vi "HFRR ADV v03.vi"() -> ()   [LabVIEW 2025] (continued)
            n967 = File Dialog(6:"*.dgf" ("pattern"), 7:w2452, 11:w2437) -> (0:w2435:errorcluster, 3:w2443:path)  [unwired: 4 in, 2 out]
            n968 = Unbundle(w2435) -> ()  [unwired: 3 out]
            n969 = Path To String(path=w2443) -> (string=w2438:string)
            "string1 4" <- w2438
            n970 = Match Pattern(string=w2438, regular expression=".dgf" ("substring (\"\")")) -> (before substring=w2448:string)  [unwired: 1 in, 3 out]
            n971 = Concatenate Strings(w2448, ".duf" ("Substring")) -> (w2445:string)
            n972 = String To Path(string=w2445) -> (path=w2449:path)
            n973 = call <vilib>:"Read Characters From File.vi"("file path (dialog if empty)"=w2449, "start of read offset (chars.:0)"=60 ("start of read offset (chars.: 0)")) -> ("character string"=→"String Control 8":string)  [unwired: 4 in, 3 out]
            n974 = Strip Path(path=w2443) -> (name=w2441:string)  [unwired: 1 out]
            n975 = Match Pattern(string=w2441, regular expression=".dgf") -> (before substring=→"String Control 7":string)  [unwired: 1 in, 3 out]
          }
        }
        n976 = case shown="True" "OPEN 3" {
          frame False {
          }
          frame True {
            (unwired) 0  # existing file
            w2434 = "Choose a datalog file to open"  # prompt
            n977 = local write "OPEN 3"(FALSE ("OPEN 1")) -> ()
            n978 = String To Path(string="C:\\LAB-IQ-NXT\\Data\\") -> (path=w2419:path)
            n979 = File Dialog(6:"*.dgf" ("pattern"), 7:w2434, 11:w2419) -> (0:w2417:errorcluster, 3:w2425:path)  [unwired: 4 in, 2 out]
            n980 = Unbundle(w2417) -> ()  [unwired: 3 out]
            n981 = Path To String(path=w2425) -> (string=w2420:string)
            "string1 3" <- w2420
            n982 = Match Pattern(string=w2420, regular expression=".dgf" ("substring (\"\")")) -> (before substring=w2430:string)  [unwired: 1 in, 3 out]
            n983 = Concatenate Strings(w2430, ".duf" ("Substring")) -> (w2427:string)
            n984 = String To Path(string=w2427) -> (path=w2431:path)
            n985 = call <vilib>:"Read Characters From File.vi"("file path (dialog if empty)"=w2431, "start of read offset (chars.:0)"=60 ("start of read offset (chars.: 0)")) -> ("character string"=→"String Control 6":string)  [unwired: 4 in, 3 out]
            n986 = Strip Path(path=w2425) -> (name=w2423:string)  [unwired: 1 out]
            n987 = Match Pattern(string=w2423, regular expression=".dgf") -> (before substring=→"String Control 5":string)  [unwired: 1 in, 3 out]
          }
        }
        n988 = case shown="True" "OPEN 2" {
          frame False {
          }
          frame True {
            (unwired) 0  # existing file
            w2416 = "Choose a datalog file to open"  # prompt
            n989 = local write "OPEN 2"(FALSE ("OPEN 1")) -> ()
            n990 = String To Path(string="C:\\LAB-IQ-NXT\\Data\\") -> (path=w2401:path)
            n991 = File Dialog(6:"*.dgf" ("pattern"), 7:w2416, 11:w2401) -> (0:w2399:errorcluster, 3:w2407:path)  [unwired: 4 in, 2 out]
            n992 = Unbundle(w2399) -> ()  [unwired: 3 out]
            n993 = Path To String(path=w2407) -> (string=w2402:string)
            "string1 2" <- w2402
            n994 = Match Pattern(string=w2402, regular expression=".dgf" ("substring (\"\")")) -> (before substring=w2413:string)  [unwired: 1 in, 3 out]
            n995 = Concatenate Strings(w2413, ".duf" ("Substring")) -> (w2410:string)
            n996 = String To Path(string=w2410) -> (path=w2408:path)
            n997 = call <vilib>:"Read Characters From File.vi"("file path (dialog if empty)"=w2408, "start of read offset (chars.:0)"=60 ("start of read offset (chars.: 0)")) -> ("character string"=→"String Control 4":string)  [unwired: 4 in, 3 out]
            n998 = Strip Path(path=w2407) -> (name=w2405:string)  [unwired: 1 out]
            n999 = Match Pattern(string=w2405, regular expression=".dgf") -> (before substring=→"String Control 3":string)  [unwired: 1 in, 3 out]
          }
        }
        n1000 = case shown="True" "OPEN 1" {
          frame False {
          }
          frame True {
            (unwired) 0  # existing file
            w2398 = "Choose a datalog file to open"  # prompt
            n1001 = local write "OPEN 1"(FALSE ("OPEN 1")) -> ()
            n1002 = String To Path(string="C:\\LAB-IQ-NXT\\Data\\") -> (path=w2383:path)
            n1003 = File Dialog(6:"*.dgf" ("pattern"), 7:w2398, 11:w2383) -> (0:w2381:errorcluster, 3:w2389:path)  [unwired: 4 in, 2 out]
            n1004 = Unbundle(w2381) -> ()  [unwired: 3 out]
            n1005 = Path To String(path=w2389) -> (string=w2384:string)
            "string1" <- w2384
            n1006 = Match Pattern(string=w2384, regular expression=".dgf" ("substring (\"\")")) -> (before substring=w2394:string)  [unwired: 1 in, 3 out]
            n1007 = Concatenate Strings(w2394, ".duf" ("Substring")) -> (w2390:string)
            n1008 = String To Path(string=w2390) -> (path=w2395:path)
            n1009 = call <vilib>:"Read Characters From File.vi"("file path (dialog if empty)"=w2395, "start of read offset (chars.:0)"=60 ("start of read offset (chars.: 0)")) -> ("character string"=→"String Control 2":string)  [unwired: 4 in, 3 out]
            n1010 = Strip Path(path=w2389) -> (name=w2388:string)  [unwired: 1 out]
            n1011 = Match Pattern(string=w2388, regular expression=".dgf") -> (before substring=→"String Control":string)  [unwired: 1 in, 3 out]
          }
        }
        n1012 = case shown="True" "RSTV1 4" {
          frame False {
          }
          frame True {
            n1013 = property on="Stroke" class="XYGraph (strict)"("Y Scale.Display Format:Precision"=u8 2 ("Y Scale.Format & Precision:Precision")) -> ()  [unwired: 2 in, 2 out]
            n1014 = property on="Stroke" class="XYGraph (strict)"("X Scale.Range:Minimum"=0.0 ("Y Scale.Range:Maximum"), "X Scale.Range:Maximum"=75.0 ("X Scale.Range:Minimum"), "Y Scale.Range:Minimum"=0.98, "Y Scale.Range:Maximum"=1.02) -> ()  [unwired: 2 in, 2 out]
          }
        }
        n1015 = case shown="True" "rstv2" {
          frame False {
          }
          frame True {
            n1016 = property on="Coefficient Of Friction" class="XYGraph (strict)"("X Scale.Range:Minimum"=0.0 ("Y Scale.Range:Maximum"), "X Scale.Range:Maximum"=75.0, "Y Scale.Range:Minimum"=0.0, "Y Scale.Range:Maximum"=1.0 ("X Scale.Range:Minimum")) -> ()  [unwired: 2 in, 2 out]
            n1017 = property on="Coefficient Of Friction" class="XYGraph (strict)"("Y Scale.Display Format:Precision"=u8 3 ("Y Scale.Format & Precision:Precision")) -> ()  [unwired: 2 in, 2 out]
          }
        }
        n1018 = case shown="True" "RSTV1 3" {
          frame False {
          }
          frame True {
            n1019 = property on="Air Temperature" class="XYGraph (strict)"("X Scale.Range:Minimum"=0.0 ("Y Scale.Range:Minimum"), "X Scale.Range:Maximum"=75.0 ("Y Scale.Range:Maximum"), "Y Scale.Range:Minimum"=20.0 ("X Scale.Range:Minimum"), "Y Scale.Range:Maximum"=26.0 ("X Scale.Range:Maximum")) -> ()  [unwired: 2 in, 2 out]
            n1020 = property on="Air Temperature" class="XYGraph (strict)"("Y Scale.Display Format:Precision"=u8 2 ("Y Scale.Format & Precision:Precision")) -> ()  [unwired: 2 in, 2 out]
          }
        }
        n1021 = case shown="True" "RST CP" {
          frame False {
          }
          frame True {
            n1022 = property on="Sample Temperature" class="XYGraph (strict)"("X Scale.Range:Minimum"=0.0, "X Scale.Range:Maximum"=75.0, "Y Scale.Range:Minimum"=58.0, "Y Scale.Range:Maximum"=62.0) -> ()  [unwired: 2 in, 2 out]
            n1023 = property on="Sample Temperature" class="XYGraph (strict)"("Y Scale.Display Format:Precision"=u8 2 ("Y Scale.Format & Precision:Precision")) -> ()  [unwired: 2 in, 2 out]
          }
        }
        n1024 = case shown="True" "RST CP 2" {
          frame False {
          }
          frame True {
            n1025 = property on="XY Graph 13" class="XYGraph (strict)"("X Scale.Range:Minimum"=0.0, "X Scale.Range:Maximum"=75.0, "Y Scale.Range:Minimum"=0.0, "Y Scale.Range:Maximum"=100.0) -> ()  [unwired: 2 in, 2 out]
            n1026 = property on="XY Graph 13" class="XYGraph (strict)"("Y Scale.Display Format:Precision"=u8 0 ("Y Scale.Format & Precision:Precision")) -> ()  [unwired: 2 in, 2 out]
          }
        }
        n1027 = case shown="True" "RSTV1 2" {
          frame False {
          }
          frame True {
            n1028 = property on="Humidity" class="XYGraph (strict)"("X Scale.Range:Minimum"=0.0, "X Scale.Range:Maximum"=75.0, "Y Scale.Range:Minimum"=48.0, "Y Scale.Range:Maximum"=58.0) -> ()  [unwired: 2 in, 2 out]
            n1029 = property on="Humidity" class="XYGraph (strict)"("Y Scale.Display Format:Precision"=u8 0 ("Y Scale.Format & Precision:Precision")) -> ()  [unwired: 2 in, 2 out]
          }
        }
        n1030 = case shown="True" "RST CP 3" {
          frame False {
          }
          frame True {
            n1031 = property on="Air Temp vs Rh" class="XYGraph (strict)"("X Scale.Range:Minimum"=18.0, "X Scale.Range:Maximum"=28.0 ("X Scale.Range:Minimum"), "Y Scale.Range:Minimum"=30.0 ("X Scale.Range:Minimum"), "Y Scale.Range:Maximum"=70.0 ("X Scale.Range:Minimum")) -> ()  [unwired: 2 in, 2 out]
          }
        }
      }
      frame 2 {
        # "Elapsed time\ncof\nstroke\nmean pos\nTemp\nHumidity"
        n1032 = case shown="True" "Export" {
          frame False {
          }
          frame True {
            w2583 = "                                      " ("string")
            w2585 = "\r"
            (unwired) i16 6 ("width (-)")
            w2662 = "\r"
            w2594 = "\r"
            n1033 = local read "Sample ID"() -> (w2669:string)
            n1034 = local read "Temperature after test 2"() -> (w2656:dbl)
            n1035 = local read "Test Date"() -> (w2668:string)
            n1036 = local read "String 45"() -> (w2582:string)
            n1037 = local read "String 32"() -> (w2666:string)
            n1038 = local read "String 31"() -> (w2667:string)
            n1039 = local read "String 38"() -> (w2604:string)
            n1040 = local read "Humidity after test 2"() -> (w2652:dbl)
            n1041 = local read "s.NO"() -> (w2584:string)
            n1042 = local read "String 36"() -> (w2607:string)
            n1043 = local read "Temperature before test 2"() -> (w2651:dbl)
            n1044 = local read "String 37"() -> (w2610:string)
            n1045 = local read "AVP 2"() -> (w2649:dbl)
            n1046 = local read "HCF 2"() -> (w2660:dbl)
            n1047 = local read "MWSD 2"() -> (w2648:dbl)
            n1048 = local read "String 35"() -> (w2614:string)
            n1049 = local write "Export"(FALSE ("Export")) -> ()
            n1050 = local read "Humidity before test 2"() -> (w2637:dbl)
            n1051 = Concatenate Strings("7," ("string"), w2604) -> (w2605:string)
            n1052 = Concatenate Strings("6," ("string"), w2607) -> (w2608:string)
            n1053 = local read "S 39"() -> (w2615:string)
            n1054 = Concatenate Strings("5," ("string"), w2610) -> (w2611:string)
            n1055 = local read "String 34"() -> (w2619:string)
            n1056 = Concatenate Strings("4," ("string"), w2614) -> (w2613:string)
            n1057 = Concatenate Strings("3," ("string"), w2615) -> (w2617:string)
            n1058 = local read "S 38"() -> (w2622:string)
            n1059 = Number To Fractional String(number=w2660, width (-)=i16 6, precision (6)=i16 2) -> (F-format string=w2661:string)  [unwired: 1 in]
            n1060 = Number To Fractional String(number=w2648, width (-)=i16 6, precision (6)=i16 2) -> (F-format string=w2646:string)  [unwired: 1 in]
            n1061 = Number To Fractional String(number=w2649, width (-)=i16 6, precision (6)=i16 2) -> (F-format string=w2647:string)  [unwired: 1 in]
            n1062 = Number To Fractional String(number=w2656, width (-)=i16 6, precision (6)=i16 2) -> (F-format string=w2655:string)  [unwired: 1 in]
            n1063 = Number To Fractional String(number=w2652, width (-)=i16 6, precision (6)=i16 2) -> (F-format string=w2650:string)  [unwired: 1 in]
            n1064 = Number To Fractional String(number=w2651, width (-)=i16 6, precision (6)=i16 2) -> (F-format string=w2657:string)  [unwired: 1 in]
            n1065 = Number To Fractional String(number=w2637, width (-)=i16 6, precision (6)=i16 2) -> (F-format string=w2636:string)  [unwired: 1 in]
            n1066 = local read "String 39"() -> (w2601:string)
            n1067 = Concatenate Strings("2," ("string"), w2619) -> (w2618:string)
            n1068 = local read "WS1.4 2"() -> (w2664:dbl)
            n1069 = Concatenate Strings(w2594, "," ("string"), w2582, w2584, w2583, w2666, w2669, w2583, w2667, w2668, w2594) -> (w2592:string)
            n1070 = Concatenate Strings("1," ("string"), w2622) -> (w2621:string)
            n1071 = Concatenate Strings("8," ("string"), w2601) -> (w2602:string)
            n1072 = Number To Fractional String(number=w2664, precision (6)=i16 2) -> (F-format string=w2665:string)  [unwired: 2 in]
            n1073 = Concatenate Strings(w2662, w2621, w2636, w2662, w2618, w2657, w2662, w2617, w2650, w2662, w2613, w2655, w2662, w2611, w2646, w2662, w2608, w2647, w2662, w2605, w2661, w2662, w2602, w2665) -> (w2624:string)
            n1074 = Concatenate Strings("S.No," ("string"), "                                       Parameters" ("string")) -> (w2595:string)
            n1075 = local read "TITTLE"() -> (w2590:string)
            n1076 = local read "String 33"() -> (w2599:string)
            n1077 = local read "Tested by"() -> (w2598:string)
            n1078 = Concatenate Strings("=" ("string"), w2590) -> (w2589:string)
            n1079 = local read "String 29"() -> (w2631:string)
            n1080 = Concatenate Strings("," ("string"), "                                                                             " ("string")) -> (w2587:string)
            n1081 = Concatenate Strings(w2589, w2585, w2592, w2585, w2595, w2624, w2585, w2587, w2599, w2598) -> (→"export":string)
            n1082 = Match Pattern(string=w2631, regular expression=".dwm") -> (before substring=w2627:string)  [unwired: 1 in, 3 out]
            "before substring" <- w2627
            n1083 = case shown="\"xlx\"" "Select File Type" {
              tunnel: w2627 -> [w2672 w2674 w2676]
              tunnel: [w2670 w2675 w2677] -> w2626
              frame "xlx" {
                n1084 = Concatenate Strings(w2672, ".xls" ("string")) -> (w2670:string)
              }
              frame "csv" {
                n1085 = Concatenate Strings(w2674, ".csv" ("string")) -> (w2675:string)
              }
              frame "txt" {
                n1086 = Concatenate Strings(w2676, ".txt" ("string")) -> (w2677:string)
              }
            }
            n1087 = String To Path(string=w2626) -> (path=w2633:path)
            n1088 = local read "export"() -> (w2628:string)
            n1089 = call <vilib>:"Write Characters To File.vi"("append to file? (new file:F)"=FALSE, "character string"=w2628, "file path (dialog if empty)"=w2633) -> ()  [unwired: 2 in, 1 out]
          }
        }
        n1090 = case shown="True" "OK Button 16" {
          frame False {
          }
          frame True {
            n1091 = stacked-sequence {
              frame #0 {
                n1092 = local read "Numeric 16"() -> (w2792:i32)
                n1093 = local write "Numeric 10"(w2792) -> ()
              }
              frame #1 {
                n1094 = local read "String 29"() -> (w2796:string)
                n1095 = String To Path(string=w2796) -> (path=w2795:path)
                n1096 = local read "S.NO"() -> (→"s.NO":string)
                n1097 = Open/Create/Replace File "Open File"(file path (use dialog)=w2795) -> (refnum out=w2797:refnum<file>)  [unwired: 5 in, 2 out]
                n1098 = for {
                  N: 16 -> [_]
                  tunnel: w2797 -> [w2804]
                  i -> [w2800]
                  (unwired) TRUE ("line mode (F)")
                  n1099 = Read from Text File "Read File"(file (use dialog)=w2804) -> (text=w2798:string)  [unwired: 3 in, 3 out]
                  n1100 = Match Pattern(string=w2798, regular expression="(") -> (after substring=w2803:string)  [unwired: 1 in, 3 out]
                  n1101 = Match Pattern(string=w2803, regular expression=")") -> (before substring=w2799:string)  [unwired: 1 in, 3 out]
                  n1102 = case shown="1" w2800 {
                    tunnel: w2799 -> [w2805 w2806 _ _ w2807 w2808 w2809 w2811 w2813 w2815 w2817 w2819 w2821 w2823 _]
                    tunnel: w2798 -> [_ _ _ _ _ _ _ _ _ _ _ _ _ _ _]
                    frame 0 {
                      "TITTLE" <- w2805
                    }
                    frame 1 {
                      "Sample ID" <- w2806
                    }
                    frame 2 {
                    }
                    frame 3 {
                    }
                    frame 4 {
                      "Test Date" <- w2807
                    }
                    frame 5 {
                      "Tested by" <- w2808
                    }
                    frame 6 {
                      n1103 = Fract/Exp String To Number(string=w2809) -> (number=→"Humidity before test 2":dbl)  [unwired: 3 in, 1 out]
                    }
                    frame 7 {
                      n1104 = Fract/Exp String To Number(string=w2811) -> (number=→"Temperature before test 2":dbl)  [unwired: 3 in, 1 out]
                    }
                    frame 8 {
                      n1105 = Fract/Exp String To Number(string=w2813) -> (number=→"Humidity after test 2":dbl)  [unwired: 3 in, 1 out]
                    }
                    frame 9 {
                      n1106 = Fract/Exp String To Number(string=w2815) -> (number=→"Temperature after test 2":dbl)  [unwired: 3 in, 1 out]
                    }
                    frame 10 {
                      n1107 = Fract/Exp String To Number(string=w2817) -> (number=→"MWSD 2":dbl)  [unwired: 3 in, 1 out]
                    }
                    frame 11 {
                      n1108 = Fract/Exp String To Number(string=w2819) -> (number=→"AVP 2":dbl)  [unwired: 3 in, 1 out]
                    }
                    frame 12 {
                      n1109 = Fract/Exp String To Number(string=w2821) -> (number=→"HCF 2":dbl)  [unwired: 3 in, 1 out]
                    }
                    frame 13 {
                      n1110 = Fract/Exp String To Number(string=w2823) -> (number=→"WS1.4 2":dbl)  [unwired: 3 in, 1 out]
                    }
                    frame 14, Default {
                    }
                  }
                }
              }
              frame #2 {
              }
            }
            n1111 = local write "OK Button 16"(FALSE ("OK Button 13")) -> ()
          }
        }
        n1112 = call <vilib>:"Query Available Printers.vi"() -> ("system configured printers"=w2467:string[])  [unwired: 9 in, 2 out]
        "System Configured Printers 2" <- w2467
        n1113 = Index Array(array=w2467, index="Select Printer 3") -> (element=w2469:string)
        "Selected Printer" <- w2469
        n1114 = local read "OK Button 16"() -> (w2463:bool)
        n1115 = case shown="True" "Print" {
          tunnel: w2469 -> [_ w2761]
          frame False {
          }
          frame True {
            (unwired) i16 6 ("width (-)")
            (unwired) "TESTED BY : "
            (unwired) "TESTED DATE :"
            (unwired) "SAMPLE ID : "
            (unwired) "SAMPLE DESIGN : "
            w2719 = "\r"
            w2736 = "\r"
            # "add image"
            n1116 = local read "String 45"() -> (w2679:string)
            n1117 = local read "Sample ID"() -> (w2709:string)
            n1118 = local read "Tested by"() -> (w2712:string)
            n1119 = local read "Test Date"() -> (w2710:string)
            n1120 = local read "String 32"() -> (w2714:string)
            n1121 = local read "String 31"() -> (w2713:string)
            n1122 = local read "String 33"() -> (w2715:string)
            n1123 = local read "s.NO"() -> (w2680:string)
            n1124 = call <vilib>:"New Report.vi"("report type"=enum16{"Standard Report", "HTML"}."Standard Report") -> ("report out"=w2759:refnum<class "NI_report.lvclass">, "error out"=w2758:errorcluster)  [unwired: 13 in]
            n1125 = local read "TITTLE"() -> (w2711:string)
            n1126 = call-dynamic "Set Report Header Text.vi"("report in"=w2759, "center header text"=w2711, "error in (no error)"=w2758) -> ("report out"=w2730:refnum<class "NI_report.lvclass">, "error out"=w2731:errorcluster)  [unwired: 11 in]
            n1127 = Concatenate Strings(w2736, w2679, w2680, w2736, w2714, w2709, w2736, w2713, w2710, w2736, w2715, w2712, w2736) -> (w2729:string)
            "test by" <- w2729
            n1128 = local read "Temperature after test 2"() -> (w2725:dbl)
            n1129 = local read "String 38"() -> (w2685:string)
            n1130 = local read "Humidity after test 2"() -> (w2734:dbl)
            n1131 = local read "String 36"() -> (w2689:string)
            n1132 = local read "Temperature before test 2"() -> (w2735:dbl)
            n1133 = local read "String 37"() -> (w2692:string)
            n1134 = local read "AVP 2"() -> (w2738:dbl)
            n1135 = local read "HCF 2"() -> (w2721:dbl)
            n1136 = local read "MWSD 2"() -> (w2739:dbl)
            n1137 = local read "String 35"() -> (w2694:string)
            n1138 = call-poly <vilib>:"Append Report Text.vi"("report in"=w2730, "text"=w2729, "error in (no error)"=w2731) -> ("report out"=w2733:refnum<class "NI_report.lvclass">, "error out"=w2732:errorcluster)  [unwired: 9 in, 2 out]
            n1139 = local read "Humidity before test 2"() -> (w2750:dbl)
            n1140 = Concatenate Strings("7)" ("string"), w2685) -> (w2686:string)
            n1141 = local read "S 39"() -> (w2697:string)
            n1142 = local read "String 34"() -> (w2699:string)
            n1143 = Concatenate Strings("6)" ("string"), w2689) -> (w2688:string)
            n1144 = Concatenate Strings("5)" ("string"), w2692) -> (w2691:string)
            n1145 = Concatenate Strings("4)" ("string"), w2694) -> (w2695:string)
            n1146 = Concatenate Strings("3)" ("string"), w2697) -> (w2698:string)
            n1147 = local read "S 38"() -> (w2704:string)
            n1148 = Concatenate Strings("2)" ("string"), w2699) -> (w2700:string)
            n1149 = Number To Fractional String(number=w2721, width (-)=i16 6, precision (6)=i16 2) -> (F-format string=w2720:string)  [unwired: 1 in]
            n1150 = Number To Fractional String(number=w2739, width (-)=i16 6, precision (6)=i16 2) -> (F-format string=w2741:string)  [unwired: 1 in]
            n1151 = Number To Fractional String(number=w2738, width (-)=i16 6, precision (6)=i16 2) -> (F-format string=w2740:string)  [unwired: 1 in]
            n1152 = Number To Fractional String(number=w2725, width (-)=i16 6, precision (6)=i16 2) -> (F-format string=w2726:string)  [unwired: 1 in]
            n1153 = Number To Fractional String(number=w2734, width (-)=i16 6, precision (6)=i16 2) -> (F-format string=w2737:string)  [unwired: 1 in]
            n1154 = Number To Fractional String(number=w2735, width (-)=i16 6, precision (6)=i16 2) -> (F-format string=w2724:string)  [unwired: 1 in]
            n1155 = Number To Fractional String(number=w2750, width (-)=i16 6, precision (6)=i16 2) -> (F-format string=w2755:string)  [unwired: 1 in]
            n1156 = call-poly <vilib>:"Append Report Text.vi"("report in"=w2733, "error in (no error)"=w2732) -> ("report out"=w2754:refnum<class "NI_report.lvclass">, "error out"=w2752:errorcluster)  [unwired: 10 in, 2 out]
            n1157 = local read "String 39"() -> (w2682:string)
            n1158 = local read "WS1.4 2"() -> (w2717:dbl)
            n1159 = Concatenate Strings("1)" ("string"), w2704) -> (w2703:string)
            n1160 = Concatenate Strings("8)" ("string"), w2682) -> (w2683:string)
            n1161 = Number To Fractional String(number=w2717, precision (6)=i16 2) -> (F-format string=w2716:string)  [unwired: 2 in]
            n1162 = Concatenate Strings(w2719, w2703, w2755, w2719, w2700, w2724, w2719, w2698, w2737, w2719, w2695, w2726, w2719, w2691, w2741, w2719, w2688, w2740, w2719, w2686, w2720, w2719, w2683, w2716) -> (w2707:string)
            "export 2" <- w2707
            n1163 = call-poly <vilib>:"Append Report Text.vi"("report in"=w2754, "text"=w2707, "error in (no error)"=w2752) -> ("report out"=w2753:refnum<class "NI_report.lvclass">, "error out"=w2751:errorcluster)  [unwired: 9 in, 2 out]
            n1164 = call-dynamic "Print Report.vi"("report in"=w2753, "printer name (default)"=w2761, "error in (no error)"=w2751) -> ("report out"=w2763:refnum<class "NI_report.lvclass">, "error out"=w2764:errorcluster)  [unwired: 11 in]
            n1165 = local read "test by"() -> (w2706:string)
            n1166 = local read "TITTLE"() -> (w2708:string)
            n1167 = local write "Print"(FALSE ("Print FF")) -> ()
            n1168 = call-dynamic "Dispose Report.vi"("report in"=w2763, "error in (no error)"=w2764) -> ()  [unwired: 13 in, 1 out]
            n1169 = Concatenate Strings(w2708, w2707, w2706) -> (→"output":string)
          }
        }
        n1170 = case shown="True" w2463 {
          frame False {
          }
          frame True {
            n1171 = flat-sequence {
              frame #0 {
              }
              frame #1 {
                n1172 = Wait (ms)(milliseconds to wait=u32 100) -> ()  [unwired: 1 out]
              }
              frame #2 {
                n1173 = local write "OK Button 16"(FALSE ("Print 3")) -> ()
              }
            }
          }
        }
        n1174 = case shown="True" "OK Button 17" {
          frame False {
          }
          frame True {
            (unwired) 0  # existing file
            w2778 = "Choose a datalog file to open"  # prompt
            n1175 = local read "String"() -> (w2773:string)
            n1176 = local write "OK Button 17"(FALSE ("OK Button 17")) -> ()
            n1177 = String To Path(string=w2773) -> (path=w2774:path)
            n1178 = File Dialog(6:"*.duf" ("pattern"), 7:w2778, 11:w2774) -> (0:w2765:errorcluster, 3:w2784:path)  [unwired: 4 in, 2 out]
            n1179 = Unbundle(w2765) -> ()  [unwired: 3 out]
            n1180 = Open/Create/Replace File "Open File"(file path (use dialog)=w2784) -> (refnum out=w2776:refnum<file>)  [unwired: 5 in, 2 out]
            n1181 = Path To String(path=w2784) -> (string=w2767:string)
            n1182 = while {
              tunnel: w2776 -> [w2788]
              i -> [w2785]
              stop <- w2786 continue-if-true
              (unwired) TRUE ("line mode (F)")
              n1183 = local write "Numeric 16"(w2785) -> ()
              n1184 = Read from Text File "Read File"(file (use dialog)=w2788) -> (text=w2787:string)  [unwired: 3 in, 3 out]
              n1185 = String Length(string=w2787) -> (length=w2790:i32)
              n1186 = Greater?(x=w2790, y=1) -> (0:w2786:bool)
            }
            n1187 = local write "String 29"(w2767) -> ()
            n1188 = Match Pattern(string=w2767, regular expression=".dwm" ("substring (\"\")")) -> (before substring=w2768:string)  [unwired: 1 in, 3 out]
            "String Indicator 3" <- w2768
            n1189 = Search and Replace String(input string=w2767, search string=".duf", replace string=".dgf" ("replace string (\"\")")) -> (result string=→"String Indicator 4":string)  [unwired: 5 in, 3 out]
            n1190 = String To Path(string=w2768) -> (path=w2775:path)
            "path" <- w2775
            n1191 = Strip Path(path=w2784) -> (name=w2782:string)  [unwired: 1 out]
            n1192 = call <vilib>:"Read Characters From File.vi"("file path (dialog if empty)"=w2775, "start of read offset (chars.:0)"=60 ("start of read offset (chars.: 0)")) -> ("character string"=→"String Indicator 2":string)  [unwired: 4 in, 3 out]
            n1193 = Match Pattern(string=w2782, regular expression=".dwm") -> (before substring=w2766:string)  [unwired: 1 in, 3 out]
            "String Indicator" <- w2766
            n1194 = local write "TITTLE 2"(w2766) -> ()
          }
        }
        n1195 = case shown="True" "Print 2" {
          frame False {
          }
          frame True {
            n1196 = flat-sequence {
              frame #0 {
                n1197 = local read "Ref A Test Date :"() -> (→"TITTLE 4":string)
                n1198 = local read "Sample ID"() -> (→"Sample ID  2":string)
                n1199 = local read "s.NO"() -> (→"s.NO 2":string)
                n1200 = local read "Test Date"() -> (→"Test Date 2":string)
                n1201 = local read "Tested by"() -> (→"Tested by 2":string)
                n1202 = local read "Temperature before test 3"() -> (w2487:dbl)
                n1203 = local read "Temperature before test 3"() -> (→"Temperature after test 5":dbl)
                n1204 = local read "Temperature after test 3"() -> (→"Temperature after test 4":dbl)
                n1205 = local read "Sample ID  3"() -> (→"Sample ID  6":string)
                n1206 = local read "Sample ID  4"() -> (→"Sample ID  7":string)
                n1207 = local read "Humidity before test 3"() -> (→"Humidity before test 4":dbl)
                n1208 = local read "Humidity after test 3"() -> (→"Humidity after test 4":dbl)
                n1209 = local write "Temperature before test 3"(w2487) -> ()
                n1210 = String To Path(string="C:\\LAB-IQ-NXT\\im\\Temp_resized.jpg") -> (path=w2479:path)
                "path 2" <- w2479
                n1211 = local read "image data"() -> (w2478:T8)
                n1212 = Wait (ms)(milliseconds to wait=u32 20) -> ()  [unwired: 1 out]
                n1213 = call <vilib>:"Write JPEG File.vi"("image data"=w2478, "path to JPEG file"=w2479) -> ()  [unwired: 8 in, 2 out]
                "Ref A Test Date :" <- "Ref A Test Date :"
                "Ref B Test Date :" <- "Ref B Test Date :"
                "Ref B Scar Value :" <- "Ref B Scar Value :"
                "Ref A Scar Value :" <- "Ref A Scar Value :"
              }
              frame #1 {
                (unwired) HTML_Report_Image_Alignment."MIDDLE" ("alignment (default)")
                w2515 = u16 0 items=["portrait", "landscape"] ("orientation (portrait)")
                (unwired) HTML_Report_Image_Alignment."ABSMIDDLE" ("alignment (default)")
                (unwired) "TESTED BY : "
                (unwired) "TESTED DATE :"
                (unwired) "SAMPLE ID : "
                (unwired) "SAMPLE DESIGN : "
                w2548 = "\r"
                # "add image"
                n1214 = call <vilib>:"New Report.vi"("report type"=enum16{"Standard Report", "HTML"}."HTML") -> ("report out"=w2519:refnum<class "NI_report.lvclass">, "error out"=w2517:errorcluster)  [unwired: 13 in]
                n1215 = Wait (ms)(milliseconds to wait=u32 20) -> ()  [unwired: 1 out]
                n1216 = call-dynamic "Set Report Orientation.vi"("report in"=w2519, "orientation (portrait)"=w2515, "error in (no error)"=w2517) -> ("report out"=w2518:refnum<class "NI_report.lvclass">, "error out"=w2516:errorcluster)  [unwired: 11 in]
                n1217 = for {
                  N: 5 -> [_]
                  tunnel: w2518 -> [w2569]
                  tunnel: [w2568] -> w2497
                  tunnel: w2516 -> [w2567]
                  tunnel: [w2566] -> w2496
                  n1218 = call-dynamic "Set Report Tab Width.vi"("report in"=w2569, "error in (no error)"=w2567) -> ("report out"=w2568:refnum<class "NI_report.lvclass">, "error out"=w2566:errorcluster)  [unwired: 12 in]
                }
                n1219 = local read "Sample ID  2"() -> (w2541:string)
                n1220 = local read "s.NO 2"() -> (w2540:string)
                n1221 = local read "Test Date 2"() -> (w2542:string)
                n1222 = local read "Tested by 2"() -> (w2543:string)
                n1223 = local read "String 46"() -> (w2539:string)
                n1224 = local read "String 48"() -> (w2545:string)
                n1225 = local read "String 47"() -> (w2544:string)
                n1226 = local read "String 49"() -> (w2546:string)
                n1227 = local read "TITTLE"() -> (w2514:string)
                n1228 = call-dynamic "Set Report Header Text.vi"("report in"=w2497, "center header text"=w2514, "error in (no error)"=w2496) -> ("report out"=w2535:refnum<class "NI_report.lvclass">, "error out"=w2534:errorcluster)  [unwired: 11 in]
                n1229 = for {
                  N: 1 -> [_]
                  tunnel: [w2573] -> w2521
                  tunnel: [w2572] -> w2520
                  tunnel: w2535 -> [w2571]
                  tunnel: w2534 -> [w2570]
                  n1230 = call-dynamic "New Report Line.vi"("report in"=w2571, "error in (no error)"=w2570) -> ("report out"=w2573:refnum<class "NI_report.lvclass">, "error out"=w2572:errorcluster)  [unwired: 12 in]
                }
                n1231 = for {
                  N: 2 -> [_]
                  tunnel: [w2565] -> w2527
                  tunnel: [w2564] -> w2526
                  tunnel: w2521 -> [w2563]
                  tunnel: w2520 -> [w2562]
                  n1232 = call-dynamic "New Report Line.vi"("report in"=w2563, "error in (no error)"=w2562) -> ("report out"=w2565:refnum<class "NI_report.lvclass">, "error out"=w2564:errorcluster)  [unwired: 12 in]
                }
                n1233 = Concatenate Strings(w2548, w2539, w2540, w2548, w2545, w2541, w2548, w2544, w2542, w2548, w2546, w2543, w2548) -> (→"test by 2":string)
                n1234 = for {
                  N: 25 -> [_]
                  tunnel: w2527 -> [w2561]
                  tunnel: w2526 -> [w2559]
                  tunnel: [w2560] -> w2530
                  tunnel: [w2558] -> w2529
                  n1235 = call-dynamic "Set Report Tab Width.vi"("report in"=w2561, "error in (no error)"=w2559) -> ("report out"=w2560:refnum<class "NI_report.lvclass">, "error out"=w2558:errorcluster)  [unwired: 12 in]
                }
                n1236 = control-ref of="Tab Control 9"() -> (w2525:refnum<vi>)
                n1237 = local read "Wear Scar X"() -> (w2513:dbl)
                "Length ( microns ) 2" <- w2513
                n1238 = local read "Wear Scar Y"() -> (w2512:dbl)
                "Wear Scar Y ( microns ) :" <- w2512
                n1239 = call-dynamic "Append Control Image to Report.vi"("report in"=w2530, "alignment (default)"=HTML_Report_Image_Alignment."ABSMIDDLE", "ctrl reference"=w2525, "error in (no error)"=w2529) -> ("report out"=w2524:refnum<class "NI_report.lvclass">, "error out"=w2523:errorcluster)  [unwired: 8 in, 2 out]
                n1240 = for {
                  N: 3 -> [_]
                  tunnel: [w2557] -> w2508
                  tunnel: [w2556] -> w2507
                  tunnel: w2524 -> [w2555]
                  tunnel: w2523 -> [w2554]
                  n1241 = call-dynamic "New Report Line.vi"("report in"=w2555, "error in (no error)"=w2554) -> ("report out"=w2557:refnum<class "NI_report.lvclass">, "error out"=w2556:errorcluster)  [unwired: 12 in]
                }
                n1242 = Add(x=w2513, y=w2512) -> (x+y=w2511:dbl)
                n1243 = Divide(x=w2511, y=2.0) -> (x/y=→"Mean Wear ( microns) :":dbl)
                n1244 = for {
                  N: 100 -> [_]
                  tunnel: w2508 -> [w2553]
                  tunnel: w2507 -> [w2551]
                  tunnel: [w2552] -> w2504
                  tunnel: [w2550] -> w2502
                  n1245 = call-dynamic "Set Report Tab Width.vi"("report in"=w2553, "error in (no error)"=w2551) -> ("report out"=w2552:refnum<class "NI_report.lvclass">, "error out"=w2550:errorcluster)  [unwired: 12 in]
                }
                n1246 = local read "String 10"() -> (w2499:string)
                n1247 = Concatenate Strings("C:\\LAB-IQ-NXT\\Data\\" ("string"), w2499, ".jpg" ("string")) -> ()  [unwired: 1 out]
                n1248 = String To Path(string="C:\\LAB-IQ-NXT\\im\\Temp_resized.jpg") -> (path=w2494:path)
                n1249 = call-poly <vilib>:"Append Image to Report.vi"("report in"=w2504, "path or URL of image"=w2494, "error in (no error)"=w2502) -> ("report out"=w2503:refnum<class "NI_report.lvclass">, "error out"=w2501:errorcluster)  [unwired: 9 in, 2 out]
                n1250 = call-poly <vilib>:"Open HTML Report in Browser.vi"("report in"=w2503, "error in (no error)"=w2501) -> ("report out"=w2538:refnum<class "NI_report.lvclass">, "error out"=w2537:errorcluster)  [unwired: 11 in, 1 out]
                n1251 = call-dynamic "Dispose Report.vi"("report in"=w2538, "error in (no error)"=w2537) -> ()  [unwired: 13 in, 1 out]
              }
              frame #2 {
              }
              frame #3 {
                n1252 = case shown="True" "Case Constant\n(See Context Help) 16" {
                  frame False {
                  }
                  frame True {
                    n1253 = local read "String 10"() -> (w2579:string)
                    n1254 = Concatenate Strings("C:\\LAB-IQ-NXT\\Data\\" ("string"), w2579, ".jpg" ("string")) -> (w2577:string)
                    n1255 = String To Path(string=w2577) -> (path=w2576:path)
                    n1256 = Delete(path (use dialog)=w2576) -> ()  [unwired: 4 in, 3 out]
                  }
                }
                n1257 = local write "Print 2"(FALSE ("Print")) -> ()
              }
            }
          }
        }
      }
    }
    n1258 = local read "OK Button 16"() -> (w840:bool)
    n1259 = Or(x=w840, y="OPEN") -> (x .or. y?=w841:bool)
    n1260 = case shown="True" w841 {
      tunnel: w840 -> [_ w876]
      frame False {
      }
      frame True {
        n1261 = stacked-sequence {
          tunnel: w876 -> [_ w943 _ _]
          frame #0 {
            w892 = "  " ("String 6")
            n1262 = local write "OPEN"(FALSE ("open")) -> ()
            n1263 = property on="OPEN" class="Bool (strict)"("Visible"=FALSE) -> ()  [unwired: 2 in, 2 out]
            n1264 = local write "String 12"(w892) -> ()
            n1265 = local write "String 6"(w892) -> ()
            n1266 = local write "String 7"(w892) -> ()
            n1267 = local write "String 8"(w892) -> ()
            n1268 = local read "OK Button 16"() -> (w877:bool)
            n1269 = case shown="True" w877 {
              tunnel: [w893 w894] -> w881
              frame False {
                n1270 = local read "string1"() -> (w893:string)
              }
              frame True {
                n1271 = local read "String Indicator 4"() -> (w894:string)
              }
            }
            n1272 = local read "string1 2"() -> (w880:string)
            n1273 = local read "string1 4"() -> (w878:string)
            n1274 = local read "string1 3"() -> (w879:string)
            n1275 = String To Path(string=w881) -> (path=w889:path)
            n1276 = String To Path(string=w880) -> (path=w888:path)
            n1277 = String To Path(string=w879) -> (path=w887:path)
            n1278 = String To Path(string=w878) -> (path=w886:path)
            n1279 = Open/Create/Replace File "Open File"(file path (use dialog)=w889) -> (refnum out=w885:refnum<file>)  [unwired: 5 in, 2 out]
            n1280 = Open/Create/Replace File "Open File"(file path (use dialog)=w888) -> (refnum out=w884:refnum<file>)  [unwired: 5 in, 2 out]
            n1281 = Open/Create/Replace File "Open File"(file path (use dialog)=w887) -> (refnum out=w883:refnum<file>)  [unwired: 5 in, 2 out]
            n1282 = Open/Create/Replace File "Open File"(file path (use dialog)=w886) -> (refnum out=w882:refnum<file>)  [unwired: 5 in, 2 out]
            n1283 = while {
              tunnel: w885 -> [w900]
              i -> [w896]
              stop <- w895 continue-if-true
              (unwired) TRUE ("line mode (F)")
              n1284 = Read from Text File "Read File"(file (use dialog)=w900) -> (text=w897:string)  [unwired: 3 in, 3 out]
              n1285 = local write "Numeric 8"(w896) -> ()
              n1286 = String Length(string=w897) -> (length=w899:i32)
              n1287 = Greater?(x=w899, y=1) -> (0:w895:bool)
            }
            n1288 = while {
              tunnel: w884 -> [w906]
              i -> [w902]
              stop <- w901 continue-if-true
              (unwired) TRUE ("line mode (F)")
              n1289 = Read from Text File "Read File"(file (use dialog)=w906) -> (text=w903:string)  [unwired: 3 in, 3 out]
              n1290 = local write "Numeric 11"(w902) -> ()
              n1291 = String Length(string=w903) -> (length=w905:i32)
              n1292 = Greater?(x=w905, y=1) -> (0:w901:bool)
            }
            n1293 = while {
              tunnel: w883 -> [w912]
              i -> [w908]
              stop <- w907 continue-if-true
              (unwired) TRUE ("line mode (F)")
              n1294 = Read from Text File "Read File"(file (use dialog)=w912) -> (text=w909:string)  [unwired: 3 in, 3 out]
              n1295 = local write "Numeric 12"(w908) -> ()
              n1296 = String Length(string=w909) -> (length=w911:i32)
              n1297 = Greater?(x=w911, y=1) -> (0:w907:bool)
            }
            n1298 = while {
              tunnel: w882 -> [w918]
              i -> [w914]
              stop <- w913 continue-if-true
              (unwired) TRUE ("line mode (F)")
              n1299 = Read from Text File "Read File"(file (use dialog)=w918) -> (text=w915:string)  [unwired: 3 in, 3 out]
              n1300 = local write "Numeric 13"(w914) -> ()
              n1301 = String Length(string=w915) -> (length=w917:i32)
              n1302 = Greater?(x=w917, y=1) -> (0:w913:bool)
            }
          }
          frame #1 {
            w1070 = FALSE ("ACTUAL   MERGE")
            # "Sample Temp"
            # "ECR"
            # "COF"
            # "Time\nCOF\nFF\nTemp"
            n1303 = case shown="True" w943 {
              tunnel: [w1090 w1091] -> w944
              frame False {
                n1304 = local read "string1"() -> (w1090:string)
              }
              frame True {
                n1305 = local read "String Indicator 4"() -> (w1091:string)
              }
            }
            n1306 = local read "string1 2"() -> (w989:string)
            n1307 = local read "string1 4"() -> (w987:string)
            n1308 = local read "string1 3"() -> (w988:string)
            n1309 = String To Path(string=w987) -> (path=w1081:path)
            n1310 = String To Path(string=w989) -> (path=w1087:path)
            n1311 = String To Path(string=w944) -> (path=w1075:path)
            n1312 = Open/Create/Replace File "Open File"(file path (use dialog)=w1081) -> (refnum out=w1080:refnum<file>, error out=w1079:errorcluster)  [unwired: 5 in, 1 out]
            n1313 = Open/Create/Replace File "Open File"(file path (use dialog)=w1075) -> (refnum out=w1089:refnum<file>, error out=w1088:errorcluster)  [unwired: 5 in, 1 out]
            n1314 = Open/Create/Replace File "Open File"(file path (use dialog)=w1087) -> (refnum out=w1085:refnum<file>, error out=w1084:errorcluster)  [unwired: 5 in, 1 out]
            n1315 = String To Path(string=w988) -> (path=w1086:path)
            n1316 = local read "Numeric 8"() -> (w1074:i32)
            n1317 = Open/Create/Replace File "Open File"(file path (use dialog)=w1086) -> (refnum out=w1082:refnum<file>, error out=w1083:errorcluster)  [unwired: 5 in, 1 out]
            n1318 = local read "Numeric 13"() -> (w1073:i32)
            n1319 = local read "Numeric 11"() -> (w1071:i32)
            n1320 = local read "Numeric 12"() -> (w1072:i32)
            n1321 = for {
              N: w1071 -> [_]
              tunnel: w1085 -> [w1200]
              tunnel: w1084 -> [w1199]
              tunnel: [w1189] -> w1051 mode=indexing
              tunnel: [w1187] -> w1049 mode=indexing
              tunnel: [w1188] -> w1044 mode=indexing
              tunnel: w1070 -> [_]
              tunnel: [w1181] -> w1046 mode=indexing
              tunnel: [w1177] -> w1022 mode=indexing
              tunnel: [w1173] -> w997 mode=indexing
              tunnel: [w1169] -> w978 mode=indexing
              tunnel: [w1164] -> w936 mode=indexing
              (unwired) TRUE ("line mode (F)")
              n1322 = Read from Text File "Read File"(file (use dialog)=w1200, error in=w1199) -> (text=w1165:string)  [unwired: 2 in, 3 out]
              n1323 = String Subset(string=w1165, offset (0)=0, length (rest)=14 ("length (rest)")) -> (substring=w1193:string)
              n1324 = Fract/Exp String To Number(string=w1193) -> (number=w1189:dbl)  [unwired: 3 in, 1 out]
              n1325 = local write "String 7"(w1165) -> ()
              n1326 = String Subset(string=w1165, offset (0)=15, length (rest)=9 ("length (rest)")) -> (substring=w1196:string)
              n1327 = Fract/Exp String To Number(string=w1196) -> (number=w1187:dbl)  [unwired: 3 in, 1 out]
              n1328 = String Subset(string=w1165, offset (0)=65, length (rest)=9 ("length (rest)")) -> (substring=w1182:string)
              n1329 = Fract/Exp String To Number(string=w1182) -> (number=w1185:dbl)  [unwired: 3 in, 1 out]
              n1330 = Add(x=w1185, y=0.0) -> (x+y=w1181:dbl)
              n1331 = String Subset(string=w1165, offset (0)=35, length (rest)=9 ("length (rest)")) -> (substring=w1190:string)
              n1332 = Fract/Exp String To Number(string=w1190) -> (number=w1188:dbl)  [unwired: 3 in, 1 out]
              n1333 = String Subset(string=w1165, offset (0)=45, length (rest)=9 ("length (rest)")) -> (substring=w1178:string)
              n1334 = Fract/Exp String To Number(string=w1178) -> (number=w1177:dbl)  [unwired: 3 in, 1 out]
              n1335 = String Subset(string=w1165, offset (0)=55, length (rest)=9 ("length (rest)")) -> (substring=w1176:string)
              n1336 = Fract/Exp String To Number(string=w1176) -> (number=w1173:dbl)  [unwired: 3 in, 1 out]
              n1337 = String Subset(string=w1165, offset (0)=25, length (rest)=9 ("length (rest)")) -> (substring=w1170:string)
              n1338 = Fract/Exp String To Number(string=w1170) -> (number=w1169:dbl)  [unwired: 3 in, 1 out]
              n1339 = String Subset(string=w1165, offset (0)=85, length (rest)=9 ("length (rest)")) -> (substring=w1168:string)
              n1340 = Fract/Exp String To Number(string=w1168) -> (number=w1164:dbl)  [unwired: 3 in, 1 out]
            }
            n1341 = for {
              N: w1072 -> [_]
              tunnel: w1083 -> [w1163]
              tunnel: w1082 -> [w1162]
              tunnel: [w1152] -> w1041 mode=indexing
              tunnel: [w1150] -> w1039 mode=indexing
              tunnel: [w1151] -> w1035 mode=indexing
              tunnel: w1070 -> [_]
              tunnel: [w1144] -> w1037 mode=indexing
              tunnel: [w1140] -> w1019 mode=indexing
              tunnel: [w1136] -> w995 mode=indexing
              tunnel: [w1133] -> w976 mode=indexing
              tunnel: [w1129] -> w935 mode=indexing
              (unwired) 9 ("length (rest)")
              (unwired) 9 ("length (rest)")
              (unwired) TRUE ("line mode (F)")
              n1342 = Read from Text File "Read File"(file (use dialog)=w1162, error in=w1163) -> (text=w1130:string)  [unwired: 2 in, 3 out]
              n1343 = String Subset(string=w1130, offset (0)=0, length (rest)=14 ("length (rest)")) -> (substring=w1156:string)
              n1344 = Fract/Exp String To Number(string=w1156) -> (number=w1152:dbl)  [unwired: 3 in, 1 out]
              n1345 = local write "String 8"(w1130) -> ()
              n1346 = String Subset(string=w1130, offset (0)=15, length (rest)=9 ("length (rest)")) -> (substring=w1159:string)
              n1347 = Fract/Exp String To Number(string=w1159) -> (number=w1150:dbl)  [unwired: 3 in, 1 out]
              n1348 = String Subset(string=w1130, offset (0)=65, length (rest)=9 ("length (rest)")) -> (substring=w1149:string)
              n1349 = Fract/Exp String To Number(string=w1149) -> (number=w1146:dbl)  [unwired: 3 in, 1 out]
              n1350 = Add(x=w1146, y=0.0) -> (x+y=w1144:dbl)
              n1351 = String Subset(string=w1130, offset (0)=35, length (rest)=9 ("length (rest)")) -> (substring=w1153:string)
              n1352 = Fract/Exp String To Number(string=w1153) -> (number=w1151:dbl)  [unwired: 3 in, 1 out]
              n1353 = String Subset(string=w1130, offset (0)=45, length (rest)=9 ("length (rest)")) -> (substring=w1143:string)
              n1354 = Fract/Exp String To Number(string=w1143) -> (number=w1140:dbl)  [unwired: 3 in, 1 out]
              n1355 = String Subset(string=w1130, offset (0)=55, length (rest)=9 ("length (rest)")) -> (substring=w1138:string)
              n1356 = Fract/Exp String To Number(string=w1138) -> (number=w1136:dbl)  [unwired: 3 in, 1 out]
              n1357 = String Subset(string=w1130, offset (0)=25) -> (substring=w1134:string)  [unwired: 1 in]
              n1358 = Fract/Exp String To Number(string=w1134) -> (number=w1133:dbl)  [unwired: 3 in, 1 out]
              n1359 = String Subset(string=w1130, offset (0)=85) -> (substring=w1132:string)  [unwired: 1 in]
              n1360 = Fract/Exp String To Number(string=w1132) -> (number=w1129:dbl)  [unwired: 3 in, 1 out]
            }
            n1361 = for {
              N: w1073 -> [_]
              tunnel: w1080 -> [w1128]
              tunnel: w1079 -> [w1127]
              tunnel: [w1117] -> w1033 mode=indexing
              tunnel: [w1116] -> w1026 mode=indexing
              tunnel: w1070 -> [_]
              tunnel: [w1105] -> w1031 mode=indexing
              tunnel: [w1110] -> w1028 mode=indexing
              tunnel: [w1106] -> w1018 mode=indexing
              tunnel: [w1101] -> w993 mode=indexing
              tunnel: [w1097] -> w974 mode=indexing
              tunnel: [w1092] -> w934 mode=indexing
              (unwired) 1.0 ("x")
              (unwired) TRUE ("line mode (F)")
              n1362 = Read from Text File "Read File"(file (use dialog)=w1128, error in=w1127) -> (text=w1093:string)  [unwired: 2 in, 3 out]
              n1363 = String Subset(string=w1093, offset (0)=0, length (rest)=14 ("length (rest)")) -> (substring=w1121:string)
              n1364 = Fract/Exp String To Number(string=w1121) -> (number=w1117:dbl)  [unwired: 3 in, 1 out]
              n1365 = String Subset(string=w1093, offset (0)=15, length (rest)=9 ("length (rest)")) -> (substring=w1124:string)
              n1366 = local write "String 12"(w1093) -> ()
              n1367 = Fract/Exp String To Number(string=w1124) -> (number=w1105:dbl)  [unwired: 3 in, 1 out]
              n1368 = String Subset(string=w1093, offset (0)=65, length (rest)=9 ("length (rest)")) -> (substring=w1111:string)
              n1369 = Fract/Exp String To Number(string=w1111) -> (number=w1114:dbl)  [unwired: 3 in, 1 out]
              n1370 = Add(x=w1114, y=0.0) -> (x+y=w1110:dbl)
              n1371 = String Subset(string=w1093, offset (0)=35, length (rest)=9 ("length (rest)")) -> (substring=w1118:string)
              n1372 = Fract/Exp String To Number(string=w1118) -> (number=w1116:dbl)  [unwired: 3 in, 1 out]
              n1373 = String Subset(string=w1093, offset (0)=45, length (rest)=9 ("length (rest)")) -> (substring=w1108:string)
              n1374 = Fract/Exp String To Number(string=w1108) -> (number=w1106:dbl)  [unwired: 3 in, 1 out]
              n1375 = String Subset(string=w1093, offset (0)=55, length (rest)=9 ("length (rest)")) -> (substring=w1103:string)
              n1376 = Fract/Exp String To Number(string=w1103) -> (number=w1101:dbl)  [unwired: 3 in, 1 out]
              n1377 = String Subset(string=w1093, offset (0)=25, length (rest)=9 ("length (rest)")) -> (substring=w1099:string)
              n1378 = Fract/Exp String To Number(string=w1099) -> (number=w1097:dbl)  [unwired: 3 in, 1 out]
              n1379 = String Subset(string=w1093, offset (0)=85, length (rest)=9 ("length (rest)")) -> (substring=w1095:string)
              n1380 = Fract/Exp String To Number(string=w1095) -> (number=w1092:dbl)  [unwired: 3 in, 1 out]
            }
            n1381 = for {
              N: w1074 -> [_]
              tunnel: w1089 -> [w1237]
              tunnel: w1088 -> [w1236]
              tunnel: [w1226] -> w1001 mode=indexing
              tunnel: [w1224] -> w1058 mode=indexing
              tunnel: [w1225] -> w1053 mode=indexing
              tunnel: w1070 -> [_]
              tunnel: [w1218] -> w1055 mode=indexing
              tunnel: [w1214] -> w1024 mode=indexing
              tunnel: [w1210] -> w999 mode=indexing
              tunnel: [w1206] -> w980 mode=indexing
              tunnel: [w1201] -> w940 mode=indexing
              (unwired) TRUE ("line mode (F)")
              # "freq"
              # "Stroke"
              # "Time"
              # "CoF"
              # "Humidity"
              # "Temp"
              # "Air Temp"
              # "ECR"
              n1382 = Read from Text File "Read File"(file (use dialog)=w1237, error in=w1236) -> (text=w1202:string)  [unwired: 2 in, 3 out]
              n1383 = String Subset(string=w1202, offset (0)=0, length (rest)=14 ("length (rest)")) -> (substring=w1230:string)
              n1384 = Fract/Exp String To Number(string=w1230) -> (number=w1226:dbl)  [unwired: 3 in, 1 out]
              n1385 = local write "String 6"(w1202) -> ()
              n1386 = String Subset(string=w1202, offset (0)=15, length (rest)=9 ("length (rest)")) -> (substring=w1233:string)
              n1387 = Fract/Exp String To Number(string=w1233) -> (number=w1224:dbl)  [unwired: 3 in, 1 out]
              n1388 = String Subset(string=w1202, offset (0)=65, length (rest)=9 ("length (rest)")) -> (substring=w1223:string)
              n1389 = Fract/Exp String To Number(string=w1223) -> (number=w1220:dbl)  [unwired: 3 in, 1 out]
              n1390 = Add(x=w1220, y=0.0) -> (x+y=w1218:dbl)
              n1391 = String Subset(string=w1202, offset (0)=35, length (rest)=9 ("length (rest)")) -> (substring=w1227:string)
              n1392 = Fract/Exp String To Number(string=w1227) -> (number=w1225:dbl)  [unwired: 3 in, 1 out]
              n1393 = String Subset(string=w1202, offset (0)=45, length (rest)=9 ("length (rest)")) -> (substring=w1217:string)
              n1394 = Fract/Exp String To Number(string=w1217) -> (number=w1214:dbl)  [unwired: 3 in, 1 out]
              n1395 = String Subset(string=w1202, offset (0)=55, length (rest)=9 ("length (rest)")) -> (substring=w1211:string)
              n1396 = Fract/Exp String To Number(string=w1211) -> (number=w1210:dbl)  [unwired: 3 in, 1 out]
              n1397 = String Subset(string=w1202, offset (0)=25, length (rest)=9 ("length (rest)")) -> (substring=w1209:string)
              n1398 = Fract/Exp String To Number(string=w1209) -> (number=w1206:dbl)  [unwired: 3 in, 1 out]
              n1399 = String Subset(string=w1202, offset (0)=85, length (rest)=9 ("length (rest)")) -> (substring=w1203:string)
              n1400 = Fract/Exp String To Number(string=w1203) -> (number=w1201:dbl)  [unwired: 3 in, 1 out]
            }
            n1401 = Delete From Array(array=w1041, index=0) -> (array with subset deleted=w924:dbl[])  [unwired: 1 in, 1 out]
            n1402 = Delete From Array(array=w1033, index=0) -> (array with subset deleted=w922:dbl[])  [unwired: 1 in, 1 out]
